vi "search for alias.vi"(10 "instance id":string, 11 "instance data":refnum<class "NISE_CEF_serializable configuration.lvclass">[](array[class])) -> (3 "index":i32)   [LabVIEW 2013, in "NISE_CEF_serializable configuration.lvclass"]
uses:
  serializable configuration/NISE_CEF_serializable configuration.lvclass
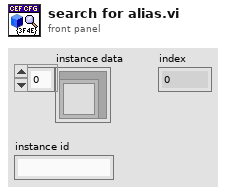
[diagram p1: front panel]
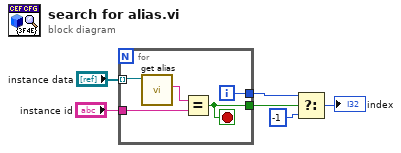
[diagram p0: block diagram]
diagram:
  n1 = for {
    tunnel: "instance data" -> [w8] mode=indexing
    tunnel: "instance id" -> [w11]
    tunnel: [w10] -> w2
    tunnel: [w9] -> w4
    i -> [w10]
    stop <- w9 stop-if-true
    n2 = call "get alias.vi"("configuration in"=w8) -> ("alias"=w7:string)  [unwired: 8 in, 2 out]
    n3 = Equal?(x=w7, y=w11) -> (x = y?=w9:bool)
  }
  n4 = Select(t=w2, s=w4, f=-1) -> (s? t:f=→"index":i32)
